vi "Script - get FrameNames.vi"(8 "error in":errorcluster, 11 "StructRef":refnum<vi>) -> (0 "error out":errorcluster, 1 "Visible Frame Index":u32, 2 "Visible Frame Name":string, 3 "Frame Names":string[](array[string]), 4 "Visible Frame":refnum<vi>, 5 "Frames[]":refnum<vi>[](array[refnum]))   [LabVIEW 2020]
uses:
  <userlib>/_OpenG.lib/string/string.llb/Trim Whitespace (String Array)__ogtk.vi
  <userlib>/_OpenG.lib/string/string.llb/openg_string.lvlib
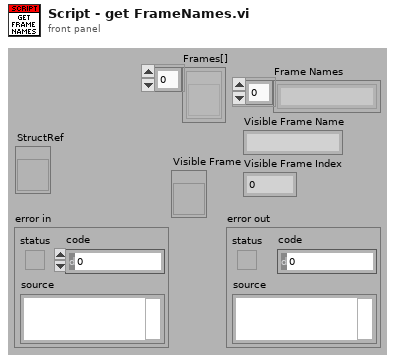
[diagram p1: front panel]
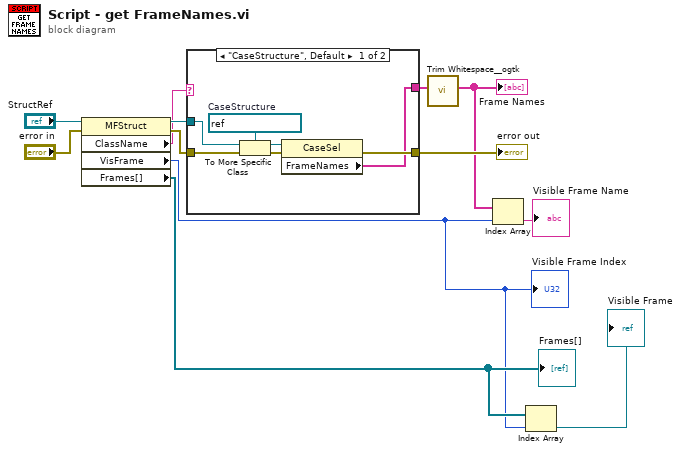
[diagram p0: block diagram]
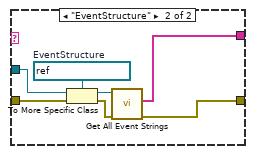
[diagram p2: hidden frame]
diagram:
  n1 = property class="MFStruct"(reference="StructRef", error in="error in") -> (reference out=w9:refnum<vi>, error out=w7:errorcluster, "ClassName"=w6:string, "VisFrame"=w2:u32, "Frames[]"=w3:refnum<vi>[])
  "Visible Frame Index" <- w2
  "Frames[]" <- w3
  n2 = case shown="\"CaseStructure\", Default" w6 {
    tunnel: w9 -> [w15 w25]
    tunnel: [w19 w22] -> w11
    tunnel: w7 -> [w18 w26]
    tunnel: [w13 w20] -> w10
    frame "CaseStructure", Default {
      w14 = refnum<vi> refnum  # CaseStructure
      n3 = To More Specific Class(target class=w14, reference=w15, error in=w18) -> (specific class reference=w16:refnum<vi>, error out=w17:errorcluster)
      n4 = property class="CaseSel"(reference=w16, error in=w17) -> (error out=w19:errorcluster, "FrameNames"=w13:string[])  [unwired: 1 out]
    }
    frame "EventStructure" {
      w24 = refnum<vi> refnum  # EventStructure
      n5 = To More Specific Class(target class=w24, reference=w25, error in=w26) -> (specific class reference=w21:refnum<vi>, error out=w23:errorcluster)
      n6 = call "Get All Event Strings.vi"("error in"=w23, "EvntStruct Ref"=w21) -> ("error out"=w22:errorcluster, "Events"=w20:string[])  [unwired: 7 in, 1 out]
    }
  }
  "error out" <- w11
  n7 = call-poly <userlib>:"Trim Whitespace__ogtk.vi"("String in"=w10) -> ("String out"=w5:string[])  [unwired: 6 in]
  "Frame Names" <- w5
  n8 = Index Array(array=w5, index=w2) -> (element=→"Visible Frame Name":string)
  n9 = Index Array(array=w3, index=w2) -> (element=→"Visible Frame":refnum<vi>)
